vi "Lifter Sequences.vi"() -> ()   [LabVIEW 2014]
panel:
  in  "Short Sequence Load":T1={"Setpoint Commands"=[enum."Setpoint 4", enum."Setpoint 3", enum."No Op", enum."Setpoint 2", enum."No Op", enum."Setpoint 3", enum."No Op", enum."No Op", enum."No Op", enum."No Op"], "Setpoint Commands Wait for Input?"=[TRUE, FALSE, FALSE, FALSE, FALSE, FALSE, FALSE, FALSE, FALSE], "Setpoint Commands Time Wait after setpoint reachd"=[0, 0, 400, 0, 300, 0, 0, 0, 300], "Can Solenoid Commands"=[enum."Disengaged", enum."Disengaged", enum."Disengaged", enum."Disengaged", enum."Disengaged", enum."Disengaged", enum."Disengaged", enum."Disengaged"], "Grabber Solenoid Commands"=[enum."Engaged", enum."Engaged", enum."Disengaged", enum."Disengaged", enum."Engaged", enum."Engaged", enum."Engaged", enum."Engaged", enum."Engaged"]}
  in  "Lift From Feeder Station WITH CAN Commands":T1={"Setpoint Commands"=[enum."Setpoint 1", enum."No Op", enum."Setpoint 5", enum."No Op", enum."No Op", enum."Setpoint 3", enum."Setpoint 2", enum."Setpoint 1", enum."No Op", enum."Setpoint 2", enum."No Op", enum."No Op", enum."Setpoint 4", enum."Setpoint 3", enum."No Op", enum."Setpoint 2", enum."No Op", enum."Setpoint 5", enum."Setpoint 3", enum."No Op", enum."Setpoint 2", enum."No Op", enum."Setpoint 5", enum."Setpoint 3", enum."No Op", enum."Setpoint 2", enum."No Op", enum."Setpoint 5", enum."Setpoint 3", enum."No Op", enum."Setpoint 2", enum."No Op", enum."Setpoint 5", enum."Setpoint 3", enum."No Op", enum."Setpoint 2", enum."No Op", enum."Setpoint 5"], "Setpoint Commands Wait for Input?"=[TRUE, FALSE, FALSE, FALSE, FALSE, FALSE, TRUE, FALSE, FALSE, TRUE, FALSE, FALSE, TRUE, FALSE, FALSE, FALSE, FALSE, TRUE, FALSE, FALSE, FALSE, FALSE, TRUE, FALSE, FALSE, FALSE, FALSE, TRUE, FALSE, FALSE, FALSE, FALSE, TRUE, FALSE, FALSE, FALSE, FALSE, TRUE, FALSE, FALSE, FALSE, FALSE, FALSE], "Setpoint Commands Time Wait after setpoint reachd"=[0, 300, 0, 300, 300, 0, 0, 0, 300, 0, 150, 150, 0, 0, 600, 0, 300, 0, 0, 600, 0, 300, 0, 0, 600, 0, 300, 0, 0, 600, 0, 300, 0, 0, 600, 0, 300, 0, 0], "Can Solenoid Commands"=[enum."Disengaged", enum."Disengaged", enum."Disengaged", enum."Engaged", enum."Engaged", enum."Engaged", enum."Engaged", enum."Engaged", enum."Engaged", enum."Engaged", enum."Engaged", enum."Engaged", enum."Engaged", enum."Disengaged", enum."Disengaged", enum."Disengaged", enum."Disengaged", enum."Disengaged", enum."Disengaged", enum."Disengaged", enum."Disengaged", enum."Disengaged", enum."Disengaged", enum."Disengaged", enum."Disengaged", enum."Disengaged", enum."Disengaged", enum."Disengaged", enum."Disengaged", enum."Disengaged", enum."Disengaged", enum."Disengaged", enum."Disengaged", enum."Disengaged", enum."Disengaged"], "Grabber Solenoid Commands"=[enum."Disengaged", enum."Engaged", enum."Engaged", enum."Engaged", enum."Disengaged", enum."Disengaged", enum."Engaged", enum."Engaged", enum."Disengaged", enum."Disengaged", enum."Disengaged", enum."Engaged", enum."Engaged", enum."Engaged", enum."Disengaged", enum."Disengaged", enum."Engaged", enum."Engaged", enum."Engaged", enum."Disengaged", enum."Disengaged", enum."Engaged", enum."Engaged", enum."Engaged", enum."Disengaged", enum."Disengaged", enum."Engaged", enum."Engaged", enum."Engaged", enum."Disengaged", enum."Disengaged", enum."Engaged", enum."Engaged", enum."Engaged", enum."Disengaged", enum."Disengaged", enum."Engaged", enum."Engaged"]}
  in  "Lift From Feeder Station NO CAN Commands":T1={"Setpoint Commands"=[enum."Setpoint 3", enum."Setpoint 2", enum."Setpoint 1", enum."No Op", enum."Setpoint 2", enum."No Op", enum."No Op", enum."Setpoint 4", enum."Setpoint 3", enum."No Op", enum."Setpoint 2", enum."No Op", enum."Setpoint 5", enum."Setpoint 3", enum."No Op", enum."Setpoint 2", enum."No Op", enum."Setpoint 5", enum."Setpoint 3", enum."No Op", enum."Setpoint 2", enum."No Op", enum."Setpoint 5", enum."Setpoint 3", enum."No Op", enum."Setpoint 2", enum."No Op", enum."Setpoint 5", enum."Setpoint 3", enum."No Op", enum."Setpoint 2", enum."No Op", enum."Setpoint 5"], "Setpoint Commands Wait for Input?"=[FALSE, TRUE, FALSE, FALSE, TRUE, FALSE, FALSE, TRUE, FALSE, FALSE, FALSE, FALSE, TRUE, FALSE, FALSE, FALSE, FALSE, TRUE, FALSE, FALSE, FALSE, FALSE, TRUE, FALSE, FALSE, FALSE, FALSE, TRUE, FALSE, FALSE, FALSE, FALSE, TRUE, FALSE, FALSE, FALSE, FALSE, FALSE], "Setpoint Commands Time Wait after setpoint reachd"=[0, 0, 0, 150, 0, 150, 150, 0, 0, 600, 0, 300, 0, 0, 600, 0, 300, 0, 0, 600, 0, 300, 0, 0, 600, 0, 300, 0, 0, 600, 0, 300, 0, 0], "Can Solenoid Commands"=[enum."Engaged", enum."Engaged", enum."Engaged", enum."Engaged", enum."Engaged", enum."Engaged", enum."Engaged", enum."Engaged"], "Grabber Solenoid Commands"=[enum."Disengaged", enum."Engaged", enum."Engaged", enum."Disengaged", enum."Disengaged", enum."Disengaged", enum."Engaged", enum."Engaged", enum."Engaged", enum."Disengaged", enum."Disengaged", enum."Engaged", enum."Engaged", enum."Engaged", enum."Disengaged", enum."Disengaged", enum."Engaged", enum."Engaged", enum."Engaged", enum."Disengaged", enum."Disengaged", enum."Engaged", enum."Engaged", enum."Engaged", enum."Disengaged", enum."Disengaged", enum."Engaged", enum."Engaged", enum."Engaged", enum."Disengaged", enum."Disengaged", enum."Engaged", enum."Engaged"]}
  in  "Drop Stack Commands":T1={"Setpoint Commands"=[enum."Setpoint 3", enum."No Op", enum."Setpoint 1", enum."No Op", enum."Setpoint 2", enum."No Op", enum."Setpoint 1", enum."No Op", enum."Setpoint 2", enum."No Op", enum."No Op", enum."No Op"], "Setpoint Commands Wait for Input?"=[FALSE, FALSE, FALSE, FALSE, FALSE, TRUE, FALSE, FALSE, FALSE], "Setpoint Commands Time Wait after setpoint reachd"=[0, 600, 0, 300, 0, 0, 0, 300, 0, 0, 0, 0], "Can Solenoid Commands"=[enum."Disengaged", enum."Disengaged", enum."Disengaged", enum."Disengaged", enum."Disengaged", enum."Engaged", enum."Disengaged", enum."Disengaged", enum."Disengaged", enum."Disengaged", enum."Disengaged", enum."Disengaged"], "Grabber Solenoid Commands"=[enum."Engaged", enum."Disengaged", enum."Disengaged", enum."Engaged", enum."Engaged", enum."Engaged", enum."Engaged", enum."Disengaged", enum."Disengaged", enum."Disengaged", enum."Disengaged", enum."Disengaged"]}
  # "WARNINGS:\n-The Sequencer uses the lifter and when it reaches setpoints as the primary method of determining when to move on to another command\n\n- Currently, giving the lifter two or more identical setpoints in a row WILL cause it to FREEZE. DO NOT INPUT MULTIPLE IDENTICAL SETPOINTS. If you need the lifter to not move for a command, use the NO OP command.\n\n- The determination of when the command Sequence is completed is when there are four (4) NO OP commands in a row. IF YOU NEED MORE THAN THREE (3) NO OP COMMANDS,SEE ZEUS AND HE WILL CHANGE THE CODE.\n\n-If there is a wait time for that command, the wait time will OVERRIDE any \"Wait for Input\". In other words, you CANNOT use a WAIT command AND a WAIT TIME command in the same command."
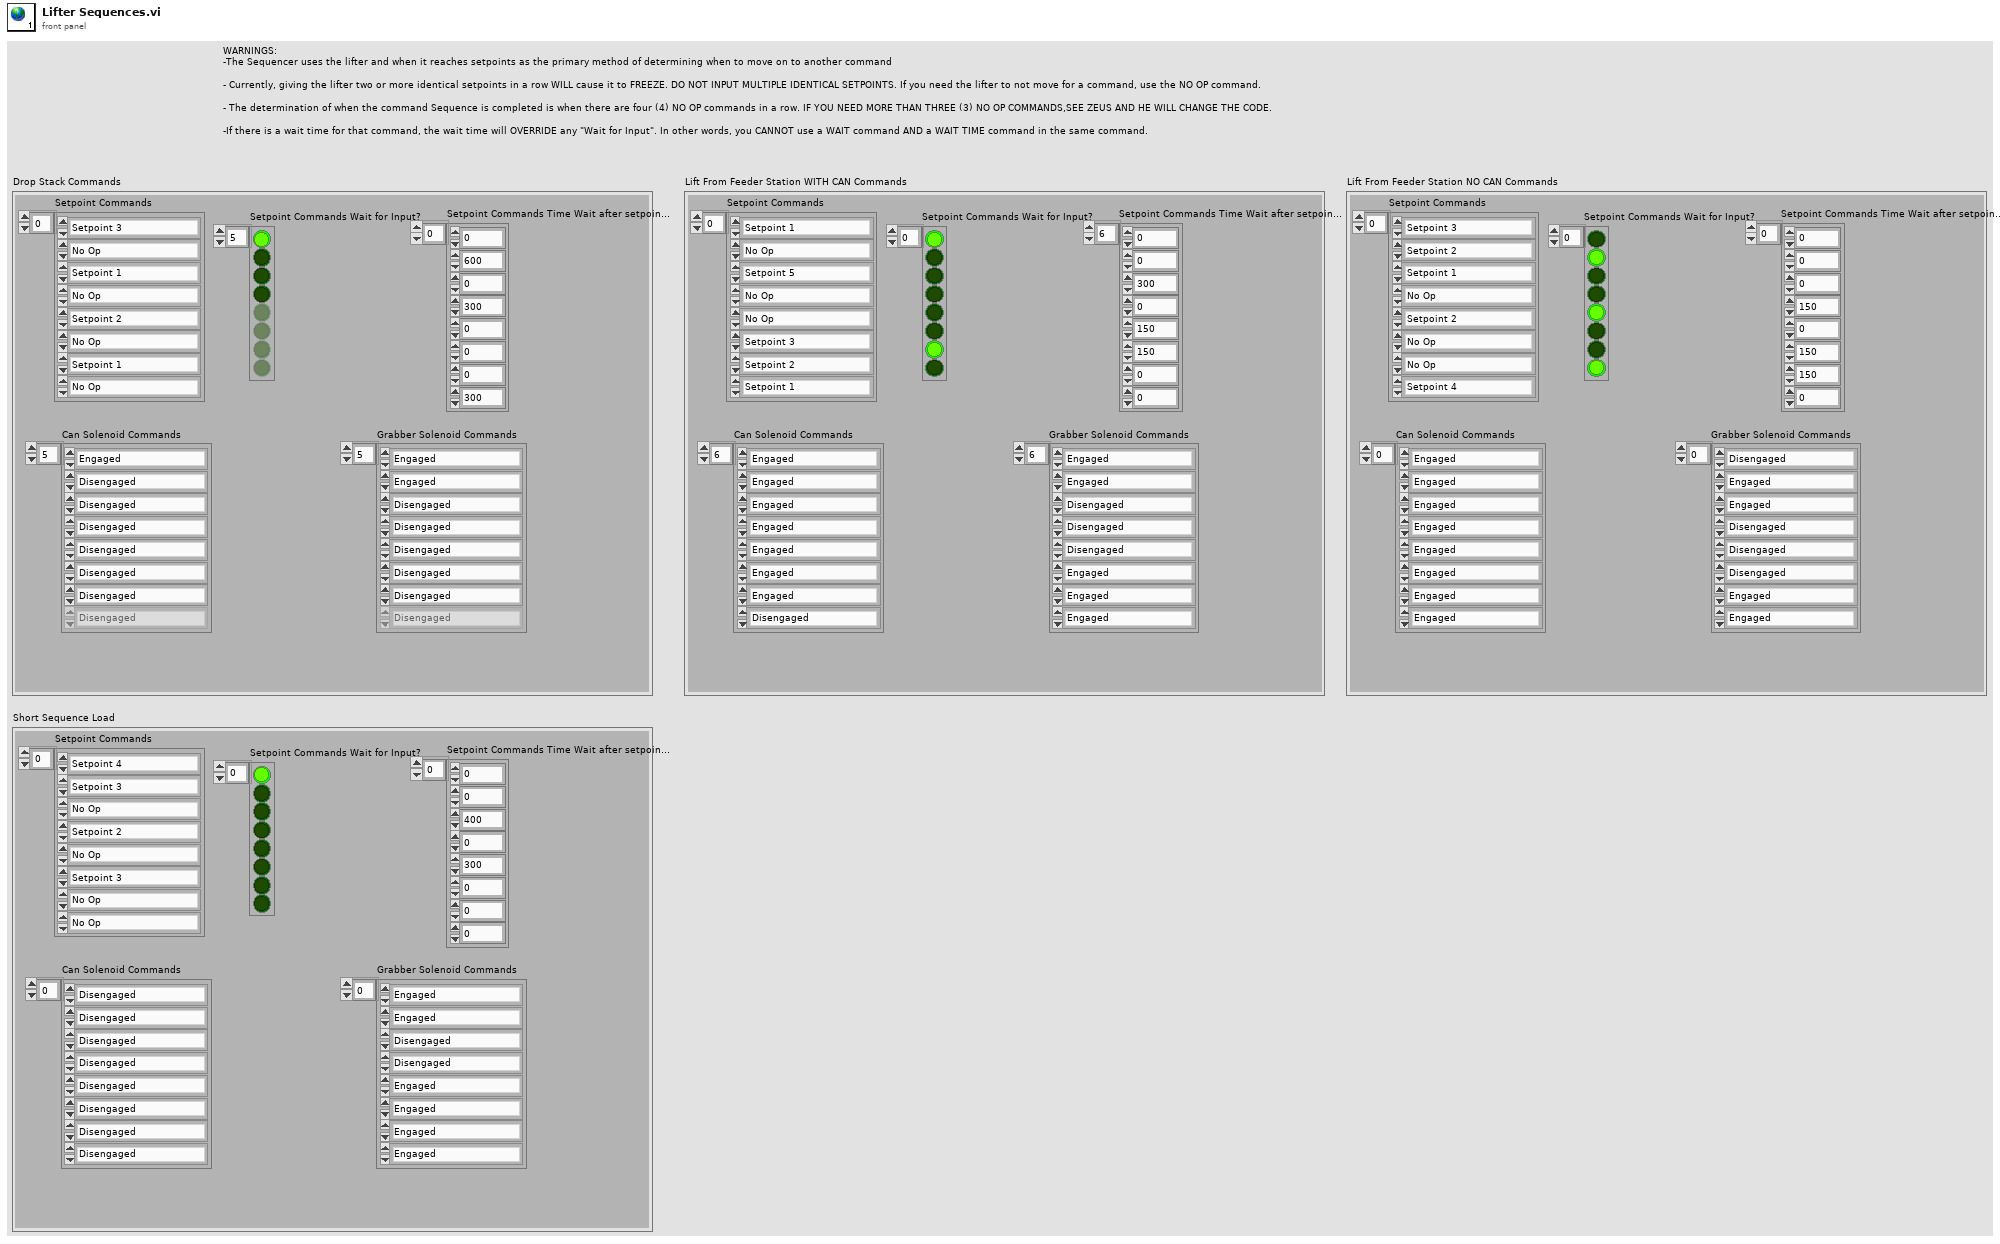
[diagram p1: front panel]
types:
  T1 = cluster{"Setpoint Commands":enum16{"No Op", "Setpoint 1", "Setpoint 2", "Setpoint 3", "Setpoint 4", "Setpoint 5"}[], "Setpoint Commands Wait for Input?":bool[], "Setpoint Commands Time Wait after setpoint reachd":i32[], "Can Solenoid Commands":enum16{"Disengaged", "Engaged"}[], "Grabber Solenoid Commands":enum16{"Disengaged", "Engaged"}[]}
diagram:
